vi "Ctor.vi"(8 "error in (no error)":errorcluster) -> (0 "error out":errorcluster, 3 "Chat Server out":refnum<class "Chat Server.lvclass">)   [LabVIEW 2012, in "Chat Server.lvclass"]
uses:
  Chat Server.lvclass
  lv-stream/stream/Connection/Connection.lvclass
  Red Data.ctl
  Stream-TCP/TCP Server/TCP Server.lvclass
  lv-stream/stream/Endpoint/Endpoint.lvclass
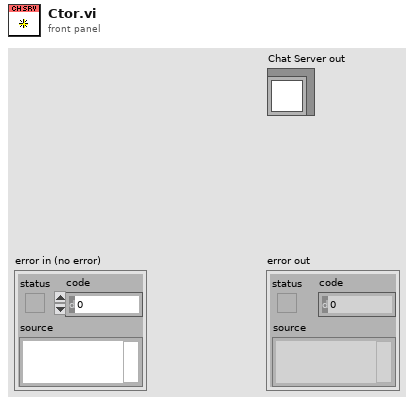
[diagram p1: front panel]
types:
  T1 = typedef "Chat Server.lvclass/Red Data.ctl" = cluster{"Connections":refnum<class "Connection.lvclass">[]}
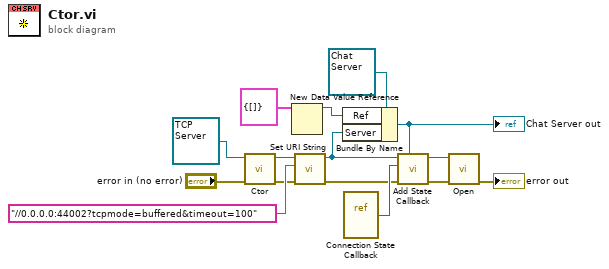
[diagram p0: block diagram]
diagram:
  n1 = call-dynamic "Ctor.vi"("error in (no error)"="error in (no error)", "TCP Server in"=refnum<class "TCP Server.lvclass"> refnum) -> ("error out"=w5:errorcluster, "TCP Server out"=w11:refnum<class "TCP Server.lvclass">)  [unwired: 8 in]
  n2 = New Data Value Reference(data value=T1 {"Connections"=[]} ("Ref Data")) -> (data value reference=w13:refnum<data-value>)  [unwired: 1 in, 1 out]
  n3 = call "Set URI String.vi"("error in (no error)"=w5, "URI String"="//0.0.0.0:44002?tcpmode=buffered&timeout=100", "Endpoint in"=w11) -> ("error out"=w4:errorcluster, "Endpoint out"=w9:refnum<class "TCP Server.lvclass">)  [unwired: 7 in]
  n4 = Bundle By Name(cluster=refnum<class "Chat Server.lvclass"> refnum ("Chat Server in"), "Ref"=w13, "Server"=w9) -> (w8:refnum<class "Chat Server.lvclass">)
  "Chat Server out" <- w8
  n5 = vi-ref "Connection State Callback.vi"() -> (w7:refnum<vi>)
  n6 = call-dynamic "Add State Callback.vi"("Owner"=w8, "error in (no error)"=w4, "Callback"=w7, "Endpoint in"=w9) -> ("error out"=w3:errorcluster, "Endpoint out"=w2:refnum<class "TCP Server.lvclass">)  [unwired: 6 in]
  n7 = call-dynamic "Open.vi"("error in (no error)"=w3, "TCP Server in"=w2) -> ("error out"=→"error out":errorcluster)  [unwired: 8 in, 1 out]
